vi "CMD_GETROT.vi"(6 "Gantry in":refnum<class "Gantry.lvclass">, 8 "error in (no error)":errorcluster, 10 "Arguments":string[](array[string]), 11 "gScript Interpreter in":refnum<class "gScript Interpreter.lvclass">) -> (0 "error out":errorcluster, 3 "gScript Interpreter out":refnum<class "gScript Interpreter.lvclass">, 4 "Gantry out":refnum<class "Gantry.lvclass">)   [LabVIEW 2017, in "gScript Interpreter.lvclass"]
uses:
  gScript Interpreter.lvclass
  Shared Components/Gantry Class/Gantry.lvclass
  Type Definitions/Memory Cell.ctl
  Type Definitions/Memory Cell Type Enum.ctl
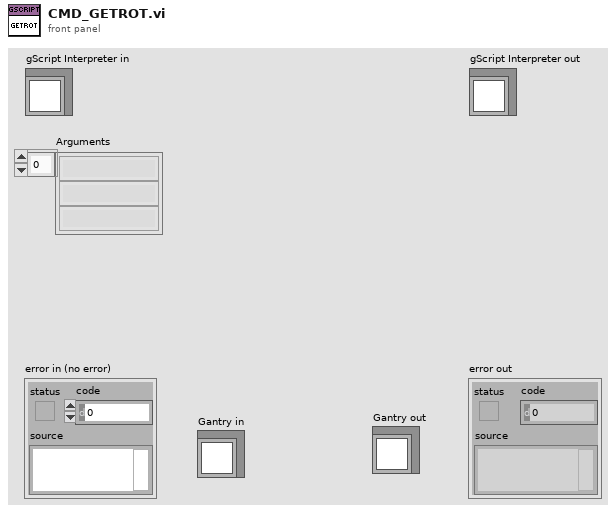
[diagram p1: front panel]
types:
  T1 = typedef "Memory Cell Type Enum.ctl" = enum16{"integer", "float", "vector", "rotation"}
  T2 = typedef "Memory Cell.ctl" = cluster{"type":T1, "x":dbl, "y":dbl, "z":dbl, "w":dbl}
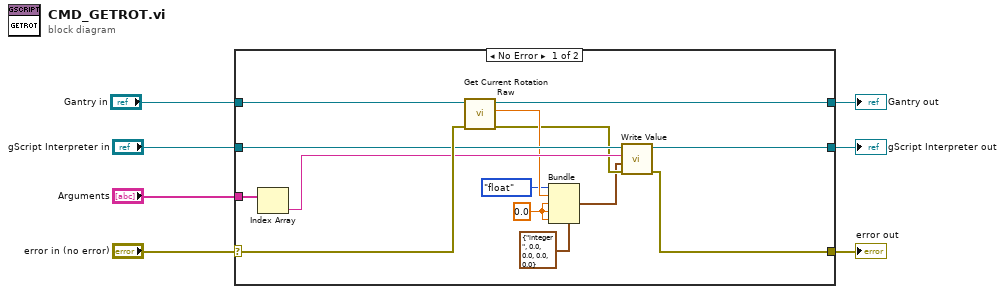
[diagram p0: block diagram]
diagram:
  n1 = case shown="No Error" "error in (no error)" {
    selector: "error in (no error)" -> [w19 w24]
    tunnel: [w8 w24] -> w6
    tunnel: [w15 w23] -> w4
    tunnel: "gScript Interpreter in" -> [w16 w23]
    tunnel: "Arguments" -> [w18 _]
    tunnel: "Gantry in" -> [w21 w22]
    tunnel: [w20 w22] -> w1
    frame No Error {
      w10 = 0.0 ("z")
      n2 = Index Array(array=w18) -> (element=w17:string)  [unwired: 1 in]
      n3 = call-dynamic "Get Current Rotation Raw.vi"("error in"=w19, "Gantry in"=w21) -> ("error out"=w12:errorcluster, "Current Rotation"=w13:dbl, "Gantry out"=w20:refnum<class "Gantry.lvclass">)  [unwired: 7 in]
      n4 = Bundle(cluster=T2 {"type"=enum."integer", "x"=0.0, "y"=0.0, "z"=0.0, "w"=0.0} ("Value"), "type"=Memory_Cell_Type_Enum."float", "x"=w13, "y"=w10, "z"=w10, "w"=w10) -> (w9:T2)
      n5 = call-dynamic "Write Value.vi"("error in (no error)"=w12, "Value"=w9, "Address"=w17, "gScript Interpreter in"=w16) -> ("error out"=w8:errorcluster, "gScript Interpreter out"=w15:refnum<class "gScript Interpreter.lvclass">)  [unwired: 6 in]
    }
    frame Error {
    }
  }
  "error out" <- w6
  "gScript Interpreter out" <- w4
  "Gantry out" <- w1
